vi "Begin.vi"(11 "Image Size":T1=enum."160x120") -> (0 "error out":errorcluster)   [LabVIEW 2011]
doc: "Called before other user functions, this VI is expected to open initial I/O refnums, load in file data, and do all program initialization. Notice that the <B>error out</B> terminal is simply used for data flow. Wiring it to other structures or subVIs ensures that this VI runs first."
uses:
  <vilib>/Rock Robotics/WPI/Camera/WPI_CameraImageSize.ctl
  <vilib>/Rock Robotics/SystemInterfaces/DIO/FPGA_DIOPWMChannel.ctl
  <vilib>/Rock Robotics/WPI/Joystick/WPI_JoystickDeviceEnum.ctl
  <vilib>/Rock Robotics/WPI/Camera/WPI_CameraWhite Balance Values.ctl
  <vilib>/Rock Robotics/WPI/Camera/WPI_CameraExposure Values.ctl
  <vilib>/Rock Robotics/WPI/Camera/WPI_CameraFrameRate.ctl
  <vilib>/Rock Robotics/WPI/Solenoid/WPI_SolenoidChannel.ctl
  <vilib>/Rock Robotics/SystemInterfaces/Typedef/FPGA_TypedefDigitalModule.ctl
  <vilib>/Rock Robotics/SystemInterfaces/DIO/FPGA_DIOChannel.ctl
  <vilib>/Rock Robotics/SystemInterfaces/DIO/FPGA_DIORelayChannel.ctl
  <vilib>/Rock Robotics/WPI/Relay/WPI_RelayDirection.ctl
  <vilib>/Rock Robotics/SystemInterfaces/Typedef/FPGA_TypedefSolenoidModule.ctl
  <vilib>/Rock Robotics/WPI/RobotDrive/WPI_RobotDriveOpen2MotorWithJaguar.vi
  <vilib>/Rock Robotics/WPI/Solenoid/WPI_SolenoidOpenDouble.vi
  <vilib>/Rock Robotics/WPI/Compressor/WPI_CompressorGetSetRefNum.vi
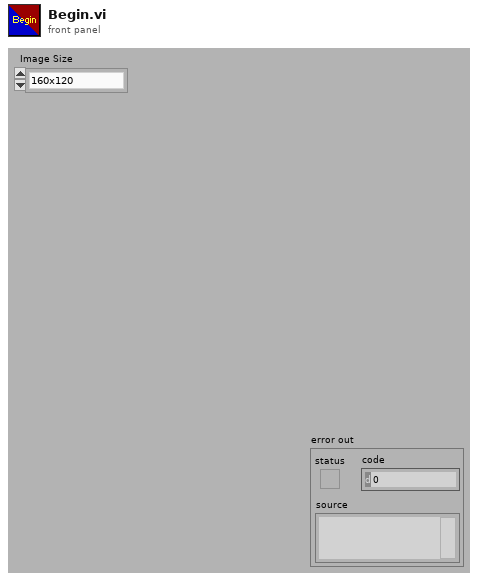
[diagram p1: front panel]
types:
  T1 = typedef "WPI_CameraImageSize.ctl" = enum16{"640x480", "320x240", "160x120"}
  T2 = typedef "WPI_RelayDirection.ctl" = enum16{"Both directions", "Forward only", "Reverse only"}
  T3 = typedef "FPGA_DIORelayChannel.ctl" = enum8{"Relay 1", "Relay 2", "Relay 3", "Relay 4", "Relay 5", "Relay 6", "Relay 7", "Relay 8", "Invalid"}
  T4 = typedef "FPGA_TypedefDigitalModule.ctl" = enum16{"Digital Module 1", "Digital Module 2"}
  T5 = typedef "WPI_SolenoidChannel.ctl" = enum8{"Solenoid 1", "Solenoid 2", "Solenoid 3", "Solenoid 4", "Solenoid 5", "Solenoid 6", "Solenoid 7", "Solenoid 8", "Invalid"}
  T6 = typedef "FPGA_TypedefSolenoidModule.ctl" = enum16{"Solenoid Module 1", "Solenoid Module 2"}
  T7 = typedef "FPGA_DIOChannel.ctl" = enum8{"DIO 1", "DIO 2", "DIO 3", "DIO 4", "DIO 5", "DIO 6", "DIO 7", "DIO 8", "DIO 9", "DIO 10", "DIO 11", "DIO 12", "DIO 13", "DIO 14", "Invalid"}
  T8 = typedef "WPI_JoystickDeviceEnum.ctl" = enum16{"USB 1", "USB 2", "USB 3", "USB 4", "Kinect 1", "Kinect 2"}
  T9 = typedef "FPGA_DIOPWMChannel.ctl" = enum8{"PWM 1", "PWM 2", "PWM 3", "PWM 4", "PWM 5", "PWM 6", "PWM 7", "PWM 8", "PWM 9", "PWM 10", "Invalid"}
  T10 = typedef "WPI_CameraFrameRate.ctl" = u32
  T11 = typedef "WPI_CameraExposure Values.ctl" = enum16{"Auto", "Flicker-free 50 Hz", "Flicker-free 60 Hz", "Hold current"}
  T12 = typedef "WPI_CameraWhite Balance Values.ctl" = enum16{"Auto", "Fixed indoor", "Fixed outdoor 1", "Fixed outdoor 2", "Fixed fluorescent 1", "Fixed fluorescent 2", "Hold current"}
  T13 = typedef "WPI_JoystickDevRef.ctl" = cluster{"Device":T8}
  T14 = typedef "WPI_CompressorDevRef.ctl" = cluster{"DevStatus":errorcluster, "DigitalInputDevRef":T15, "RelayDevRef":T16}
  T15 = typedef "WPI_DigitalInputDevRef.ctl" = cluster{"DevStatus":errorcluster, "DIO Channel":T7, "Digital Module":T4}
  T16 = typedef "WPI_RelayDevRef.ctl" = cluster{"DevStatus":errorcluster, "Relay Channel":T3, "Digital Module":T4, "Relay Direction":T2}
  T17 = typedef "WPI_CameraDevRef.ctl" = cluster{"Camera Address":string, "CameraStatus":errorcluster, "Acquire Image Notifier":refnum<notifier>}
  T18 = typedef "WPI_RobotDriveDevRef.ctl" = cluster{"DevStatus":errorcluster, "Motors[]":T19[], "Square Inputs":bool, "Max Output":dbl, "Isochronous":bool}
  T19 = typedef "WPI_MotorControlDeviceRef.ctl" = cluster{"DeviceStatus":errorcluster, "Type":enum16{"PWM", "CAN"}, "PWM":cluster{"Digital Module":T4, "PWM Channel":T9, "DeadBand":T20}, "CAN":cluster{"Device Number":u8, "Control Mode":T21, "Semaphore":T22, "Max Vout":dbl}, "Invert":bool, "TransformRef":T23, "InvTransformRef":T23}
  T20 = typedef "WPI_PWMDeadband.ctl" = cluster{"Name":string, "maxPositivePwm":i32, "minPositivePwm":i32, "centerPwm":i32, "maxNegativePwm":i32, "minNegativePwm":i32, "angularRange":u16}
  T21 = typedef "WPI_CANJaguar_ControlMode.ctl" = enum8{"Percent VBus", "Current", "Speed", "Position", "Voltage"}
  T22 = typedef "Semaphore RefNum" = refnum<k1>
  T23 = typedef "WPI_PWMTransform_ConPane.ctl" = refnum<vi>
  T24 = typedef "WPI_UltrasonicDeviceRef.ctl" = cluster{"DevStatus":errorcluster, "Ping Digital Module":T4, "Echo Digital Module":T4, "Ping Channel":T7, "Echo Channel":T7, "CntIndex":T25}
  T25 = typedef "FPGA_CounterCtrSystemIndex.ctl" = enum8{"Ctr 0", "Ctr 1", "Ctr 2", "Ctr 3", "Ctr 4", "Ctr 5", "Ctr 6", "Ctr 7", "Invalid"}
  T26 = typedef "WPI_SolenoidDevRef.ctl" = cluster{"DevStatus":errorcluster, "Solenoid Module":T6, "Forward Solenoid Channel":T5, "Reverse Solenoid Channel":T5}
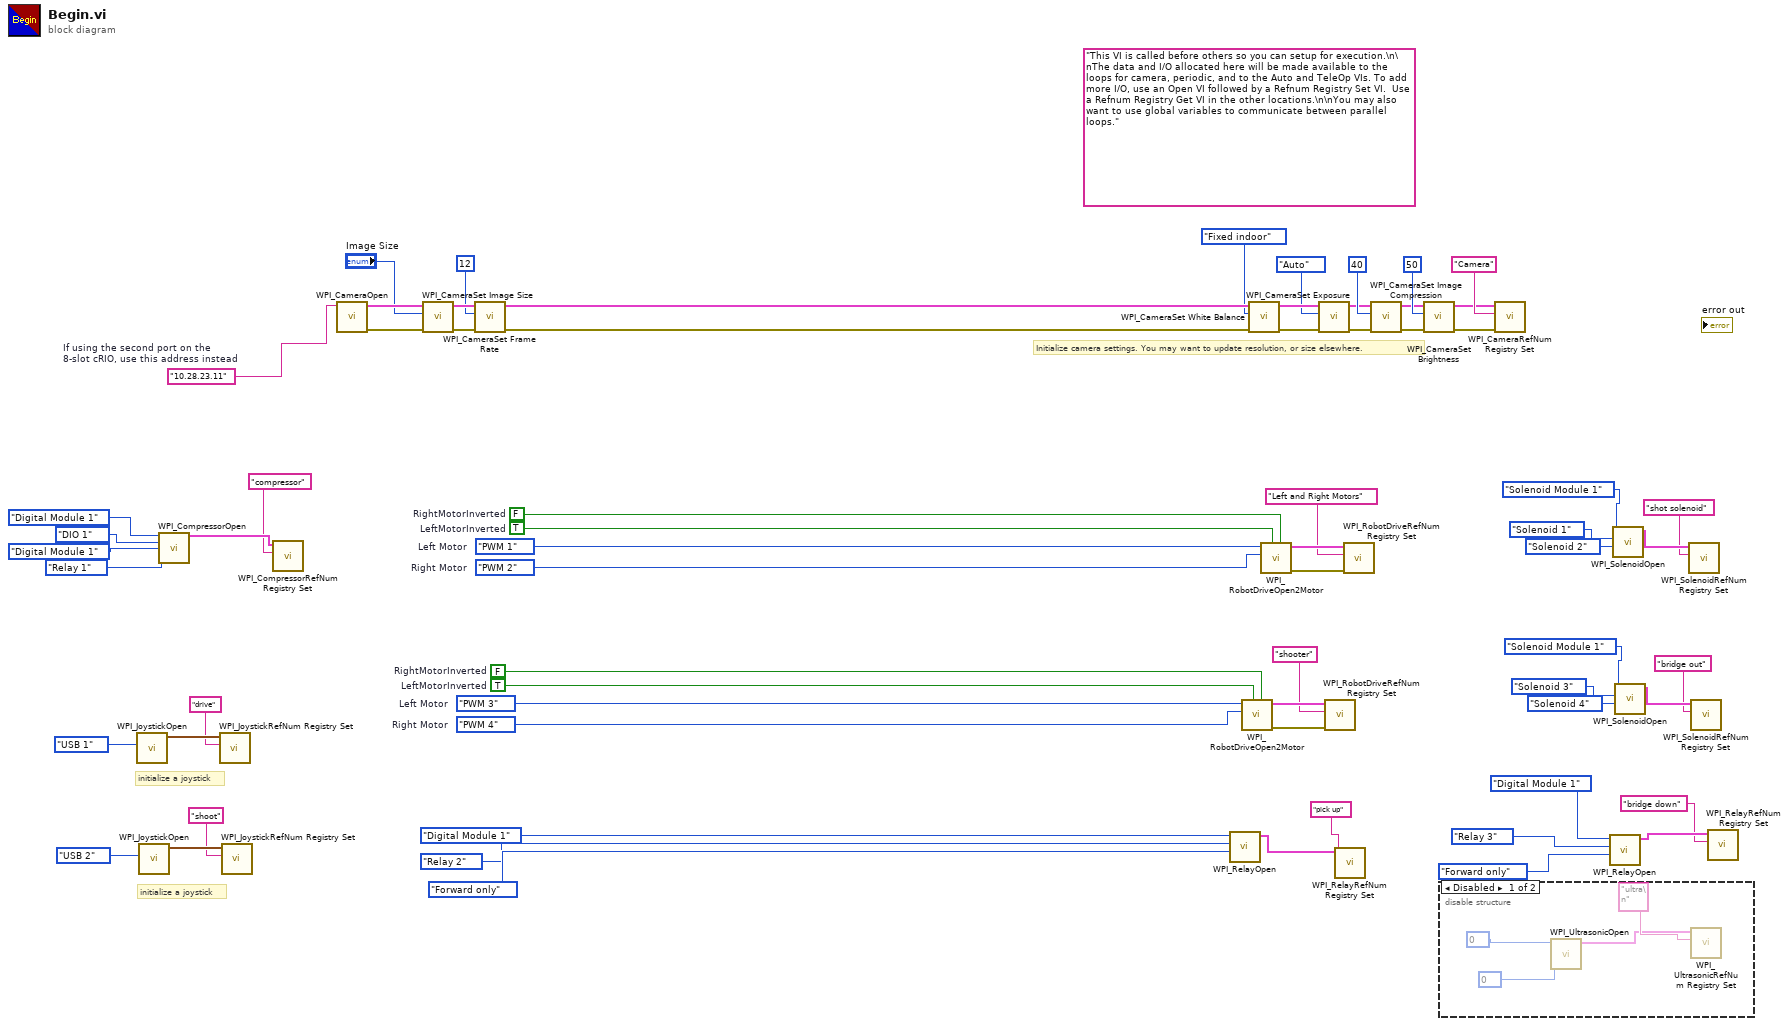
[diagram p0: block diagram]
diagram:
  w32 = FPGA_DIOPWMChannel."PWM 4"  # Right Motor
  w33 = FPGA_DIOPWMChannel."PWM 3"  # Left Motor
  w36 = TRUE  # LeftMotorInverted
  w37 = FALSE  # RightMotorInverted
  (unwired) "This VI is called before others so you can setup for execution.\n\nThe data and I/O allocated here will be made available to the loops for camera, periodic, and to the Auto and TeleOp VIs. To add more I/O, use an Open VI followed by a Refnum Registry Set VI.  Use a Refnum Registry Get VI in the other locations.\n\nYou may also want to use global variables to communicate between parallel loops."
  w42 = FPGA_DIOPWMChannel."PWM 2"  # Right Motor
  w43 = FPGA_DIOPWMChannel."PWM 1"  # Left Motor
  w1 = "10.28.23.11"  # If using the second port on the 8-slot cRIO, use this address instead
  w67 = TRUE  # LeftMotorInverted
  w68 = FALSE  # RightMotorInverted
  # "initialize a joystick"
  # "initialize a joystick"
  # "Initialize camera settings. You may want to update resolution, or size elsewhere."
  n1 = call <vilib>:"WPI_JoystickOpen.vi"("JoystickDevice"=WPI_JoystickDeviceEnum."USB 1") -> ("JoystickDevRef"=w63:T13)  [unwired: 10 out]
  n2 = call <vilib>:"WPI_JoystickOpen.vi"("JoystickDevice"=WPI_JoystickDeviceEnum."USB 2") -> ("JoystickDevRef"=w31:T13)  [unwired: 10 out]
  n3 = call <vilib>:"WPI_CompressorOpen.vi"("Pressure Switch Digital Module (Module 1)"=FPGA_TypedefDigitalModule."Digital Module 1", "Pressure Switch DIO Channel"=FPGA_DIOChannel."DIO 1", "Relay Digital Module (Module 1)"=FPGA_TypedefDigitalModule."Digital Module 1", "Relay Channel"=FPGA_DIORelayChannel."Relay 1") -> ("CompressorDevRef"=w22:T14)  [unwired: 10 in, 1 out]
  n4 = call <vilib>:"WPI_JoystickRefNum Registry Set.vi"("refnum name"="drive", "JoystickDevRef"=w63) -> ()  [unwired: 1 in, 9 out]
  n5 = call <vilib>:"WPI_JoystickRefNum Registry Set.vi"("refnum name"="shoot", "JoystickDevRef"=w31) -> ()  [unwired: 1 in, 9 out]
  n6 = call <vilib>:"WPI_CompressorRefNum Registry Set.vi"("refnum name"="compressor", "CompressorDevRef"=w22) -> ()  [unwired: 8 in, 2 out]
  n7 = call <vilib>:"WPI_CameraOpen.vi"("Camera Address"=w1) -> ("error out"=w52:errorcluster, "CameraDevRef"=w53:T17)  [unwired: 1 in, 8 out]
  n8 = call <vilib>:"WPI_CameraSet Image Size.vi"("error in (no error)"=w52, "Image Size"="Image Size", "CameraDevRef"=w53) -> ("error out"=w51:errorcluster, "CameraDevRef Out"=w54:T17)  [unwired: 7 out]
  n9 = call <vilib>:"WPI_CameraSet Frame Rate.vi"("error in (no error)"=w51, "Frame Rate (fps)"=T10 12, "CameraDevRef"=w54) -> ("error out"=w50:errorcluster, "CameraDevRef Out"=w56:T17)  [unwired: 7 out]
  n10 = call <vilib>:"WPI_RelayOpen.vi"("Relay Direction"=WPI_RelayDirection."Forward only", "Relay Channel"=FPGA_DIORelayChannel."Relay 2", "Digital Module (Module 1)"=FPGA_TypedefDigitalModule."Digital Module 1") -> ("RelayDevRef"=w16:T16)  [unwired: 7 in, 1 out]
  n11 = call-poly <vilib>:"WPI_RobotDriveOpen2Motor.vi"("Right Motor Inverted"=w37, "Left Motor Inverted"=w36, "Right Motor"=w32, "Left Motor"=w33) -> ("error out"=w34:errorcluster, "RobotDriveDevRef"=w35:T18)  [unwired: 1 in, 5 out]
  n12 = call <vilib>:"WPI_CameraSet White Balance.vi"("error in (no error)"=w50, "White Balance"=WPI_CameraWhite_Balance_Values."Fixed indoor", "CameraDevRef"=w56) -> ("error out"=w49:errorcluster, "CameraDevRef Out"=w55:T17)  [unwired: 7 out]
  n13 = call-poly <vilib>:"WPI_RobotDriveOpen2Motor.vi"("Right Motor Inverted"=w68, "Left Motor Inverted"=w67, "Right Motor"=w42, "Left Motor"=w43) -> ("error out"=w61:errorcluster, "RobotDriveDevRef"=w65:T18)  [unwired: 1 in, 5 out]
  n14 = call <vilib>:"WPI_CameraSet Exposure.vi"("error in (no error)"=w49, "Exposure"=WPI_CameraExposure_Values."Auto", "CameraDevRef"=w55) -> ("error out"=w48:errorcluster, "CameraDevRef Out"=w58:T17)  [unwired: 7 out]
  n15 = call <vilib>:"WPI_RobotDriveRefNum Registry Set.vi"("error in (no error)"=w34, "refnum name"="shooter", "RobotDriveDevRef"=w35) -> ()  [unwired: 9 out]
  n16 = call <vilib>:"WPI_RelayRefNum Registry Set.vi"("refnum name"="pick up", "RelayDevRef"=w16) -> ()  [unwired: 8 in, 2 out]
  n17 = call <vilib>:"WPI_RobotDriveRefNum Registry Set.vi"("error in (no error)"=w61, "refnum name"="Left and Right Motors", "RobotDriveDevRef"=w65) -> ()  [unwired: 9 out]
  n18 = call <vilib>:"WPI_CameraSet Image Compression.vi"("error in (no error)"=w48, "Compression"=40, "CameraDevRef"=w58) -> ("error out"=w47:errorcluster, "CameraDevRef Out"=w57:T17)  [unwired: 7 out]
  n19 = call <vilib>:"WPI_CameraSet Brightness.vi"("error in (no error)"=w47, "Brightness"=50, "CameraDevRef"=w57) -> ("error out"=w45:errorcluster, "CameraDevRef Out"=w46:T17)  [unwired: 7 out]
  n20 = disable-structure shown="Disabled" {
    frame Disabled {
      w69 = u16 0 items=[""]
      w70 = u16 0 items=[""]
      n21 = call <vilib>:"WPI_UltrasonicOpen.vi"("Echo Digital Module (Module 1)"=w69, "Ping DIO Channel"=w70) -> ("UltrasonicDevRef"=w71:T24)  [unwired: 8 in, 1 out]
      n22 = call <vilib>:"WPI_UltrasonicRefNum Registry Set.vi"("refnum name"="ultra\n", "UltrasonicDevRef"=w71) -> ()  [unwired: 8 in, 2 out]
    }
    frame Enabled {
    }
  }
  n23 = call <vilib>:"WPI_CameraRefNum Registry Set.vi"("error in (no error)"=w45, "refnum name"="Camera", "CameraDevRef"=w46) -> ()  [unwired: 9 out]
  n24 = call <vilib>:"WPI_RelayOpen.vi"("Relay Direction"=WPI_RelayDirection."Forward only", "Relay Channel"=FPGA_DIORelayChannel."Relay 3", "Digital Module (Module 1)"=FPGA_TypedefDigitalModule."Digital Module 1") -> ("RelayDevRef"=w3:T16)  [unwired: 7 in, 1 out]
  n25 = call-poly <vilib>:"WPI_SolenoidOpen.vi"("Reverse Solenoid Channel"=WPI_SolenoidChannel."Solenoid 2", "Forward Solenoid Channel"=WPI_SolenoidChannel."Solenoid 1", "Solenoid Module (Module 1)"=FPGA_TypedefSolenoidModule."Solenoid Module 1") -> ("SolenoidDevRef"=w25:T26)  [unwired: 7 in, 1 out]
  n26 = call-poly <vilib>:"WPI_SolenoidOpen.vi"("Reverse Solenoid Channel"=WPI_SolenoidChannel."Solenoid 4", "Forward Solenoid Channel"=WPI_SolenoidChannel."Solenoid 3", "Solenoid Module (Module 1)"=FPGA_TypedefSolenoidModule."Solenoid Module 1") -> ("SolenoidDevRef"=w9:T26)  [unwired: 7 in, 1 out]
  n27 = call <vilib>:"WPI_SolenoidRefNum Registry Set.vi"("refnum name"="shot solenoid", "SolenoidDevRef"=w25) -> ()  [unwired: 8 in, 2 out]
  n28 = call <vilib>:"WPI_SolenoidRefNum Registry Set.vi"("refnum name"="bridge out", "SolenoidDevRef"=w9) -> ()  [unwired: 8 in, 2 out]
  n29 = call <vilib>:"WPI_RelayRefNum Registry Set.vi"("refnum name"="bridge down", "RelayDevRef"=w3) -> ()  [unwired: 8 in, 2 out]
